vi "ClearTask.vi"(8 "error in (no error)":errorcluster, 11 "DAQ Hardware In":T1={"Task"="", "Max"=5.0, "min"=-5.0, "Samples Rate"=1000.0, "Channels"=[]} {"min" format="%0.2f"; "Max" format="%0.2f"}) -> (0 "error out":errorcluster)   [LabVIEW 2014, in "NIDAQ.lvlib"]
uses:
  NIDAQ.lvlib
  DAQHardware.ctl
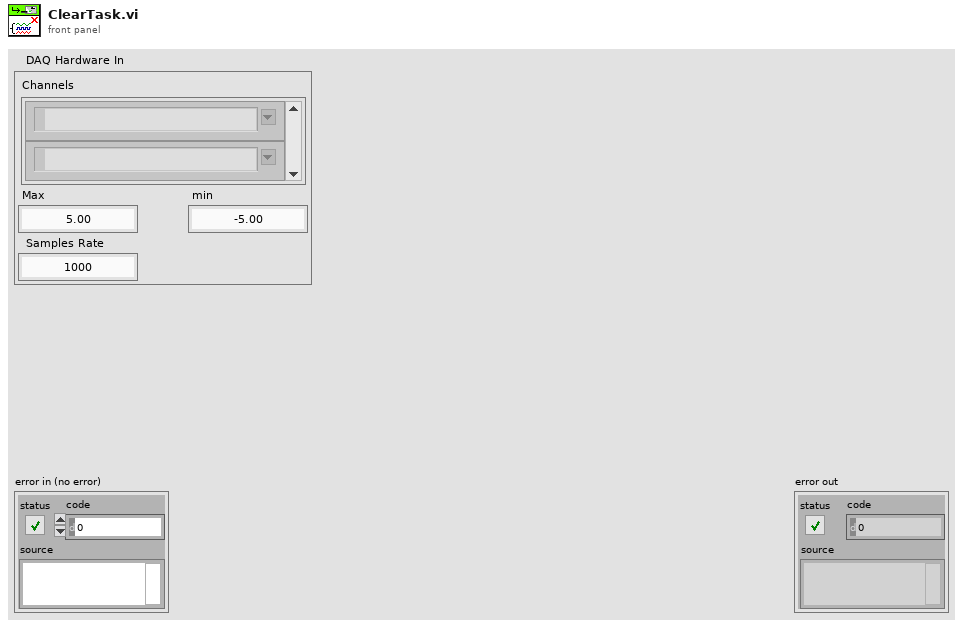
[diagram p1: front panel]
types:
  T1 = typedef "NIDAQ.lvlib/DAQHardware.ctl" = cluster{"Task":refnum<k21>, "Max":dbl, "min":dbl, "Samples Rate":dbl, "Channels":tag[]}
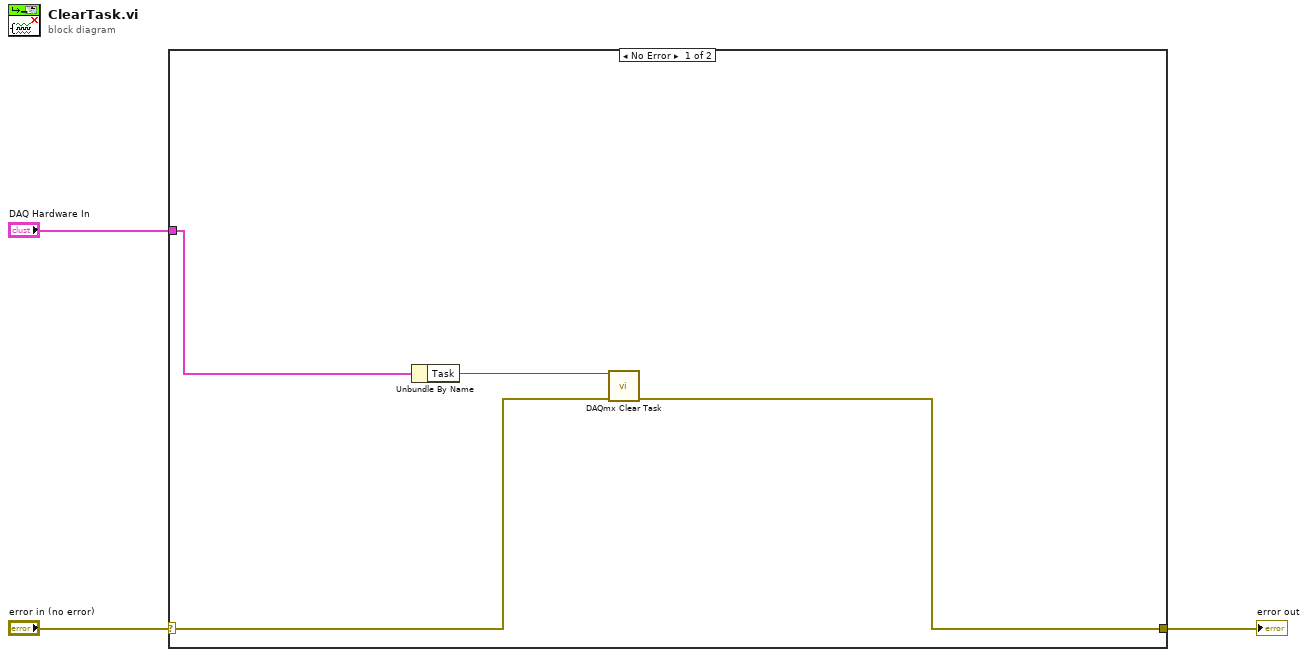
[diagram p0: block diagram]
diagram:
  n1 = case shown="No Error" "error in (no error)" {
    selector: "error in (no error)" -> [w7 w8]
    tunnel: [w6 w8] -> w2
    tunnel: "DAQ Hardware In" -> [w5 _]
    frame No Error {
      n2 = Unbundle By Name(w5) -> ("Task"=w4:refnum<k21>)
      n3 = call <vilib>:"DAQmx Clear Task.vi"("task in"=w4, "error in"=w7) -> ("error out"=w6:errorcluster)  [unwired: 13 in]
    }
    frame Error {
    }
  }
  "error out" <- w2
